vi "SetupRawDataFile.vi"(9 "Filename":string, 10 "start path":path=path "C:/Users/Eivind/Desktop/Rotation Training", 11 "Mouse Number":i32) -> (3 "TDMS storage path":path)   [LabVIEW 2013]
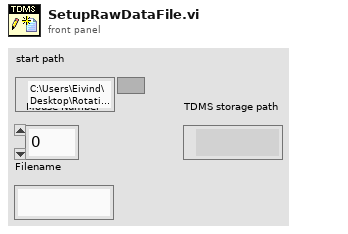
[diagram p1: front panel]
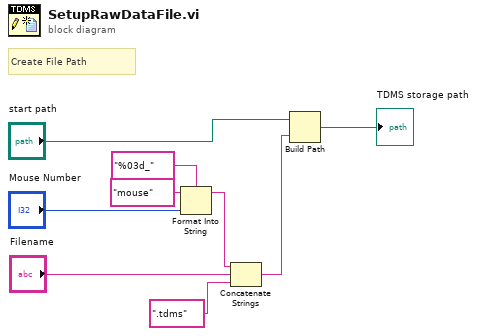
[diagram p0: block diagram]
diagram:
  # "Create File Path"
  n1 = Format Into String(format string="%03d_", initial string="mouse", "Mouse Number") -> (resulting string=w2:string)  [unwired: 1 in, 1 out]
  n2 = Concatenate Strings(w2, "Filename", ".tdms" ("string")) -> (w1:string)
  n3 = Build Path(base path="start path", name or relative path=w1) -> (appended path=→"TDMS storage path":path)
